vi "Read XML HW Configuration File_Parse Channels.vi"(8 "error in (no error)":errorcluster, 11 "channel429":refnum<k24>[](array[refnum])) -> (0 "error out":errorcluster, 3 "Array":T1[](array[typedef]) {"speed" items=["Auto", "Low", "High"]; "Labels"."scheduleBuildUnit" items=["Millisecond", "Microsecond"]})   [LabVIEW 2020]
doc: "This VI parses the XML HW DB."
uses:
  Controls/Ballard_Channel.ctl
  Controls/Ballard_Label.ctl
  Controls/Ballard_Word.ctl
  Controls/ARINCParam.ctl
  Shared/Controls and Global/TransferType.ctl
  Controls/Channel_direction.ctl
  Controls/Channel Speed.ctl
  C:/git/Ballard-Arinc-429-Custom-Device/Source/System Explorer/SubVIs/Parse XML Ballard/1.2/BTIXML_SerDes.dll
  1.2/BTIXML_SerDes.dll
  Ballard Arinc-429 System Explorer.lvlib
  Shared/Ballard Arinc-429 Shared.lvlib
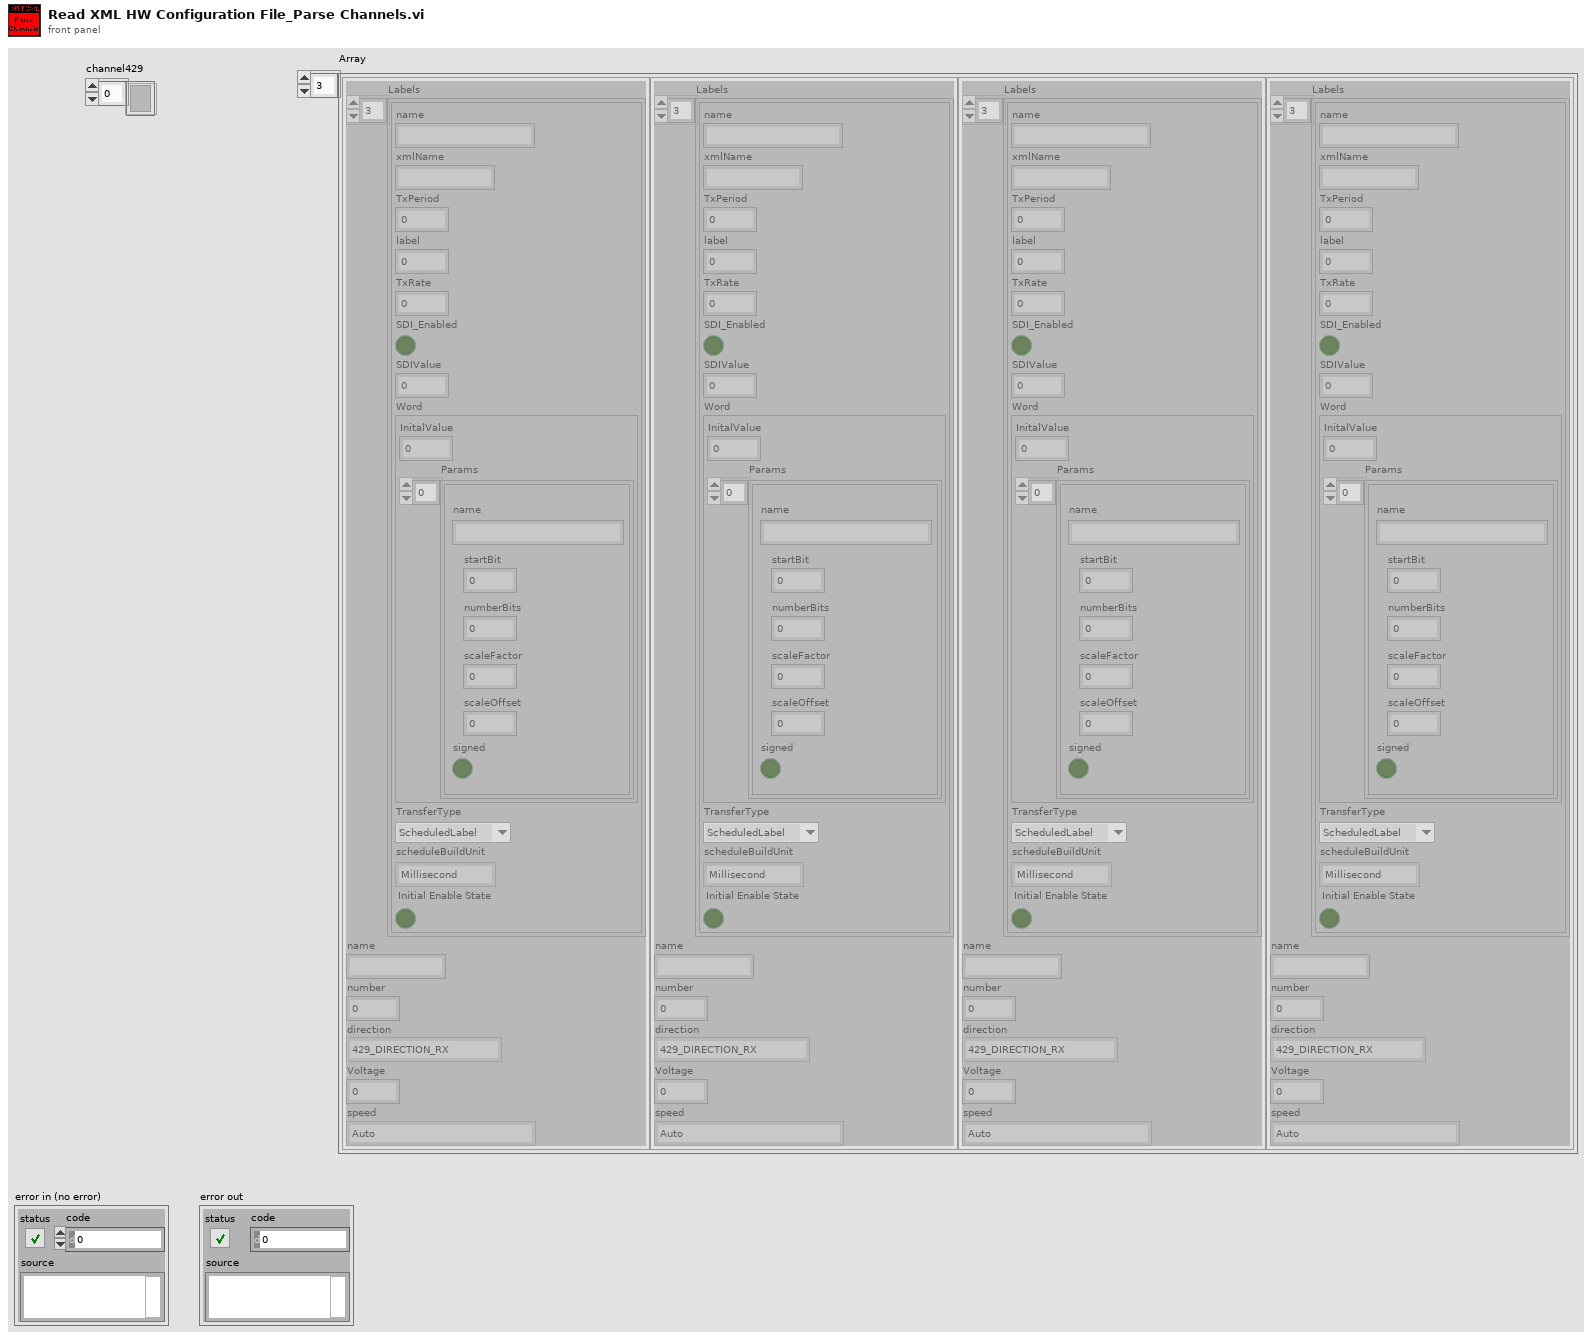
[diagram p1: front panel]
types:
  T1 = typedef "Ballard Arinc-429 System Explorer.lvlib/Ballard_Channel.ctl" = cluster{"Labels":T2[], "name":string, "number":u8, "direction":T6, "Voltage":dbl, "speed":T7}
  T2 = typedef "Ballard Arinc-429 System Explorer.lvlib/Ballard_Label.ctl" = cluster{"name":string, "xmlName":string, "TxPeriod":u32, "label":u32, "TxRate":dbl, "SDI_Enabled":bool, "SDIValue":u8, "Word":T3, "TransferType":T5, "scheduleBuildUnit":i32, "Initial Enable State":bool}
  T3 = typedef "Ballard Arinc-429 System Explorer.lvlib/Ballard_Word.ctl" = cluster{"InitalValue":u32, "Params":T4[]}
  T4 = typedef "Ballard Arinc-429 System Explorer.lvlib/ARINCParam.ctl" = cluster{"name":string, "startBit":i32, "numberBits":i32, "scaleFactor":dbl, "scaleOffset":dbl, "signed":bool}
  T5 = typedef "Ballard Arinc-429 Shared.lvlib/TransferType.ctl" = enum16{"ScheduledLabel", "Acyclic", "Block", "Strobe"}
  T6 = typedef "Ballard Arinc-429 System Explorer.lvlib/Channel_direction.ctl" = enum16{"429_DIRECTION_RX", "429_DIRECTION_TX"}
  T7 = typedef "Ballard Arinc-429 System Explorer.lvlib/Channel Speed.ctl" = i32
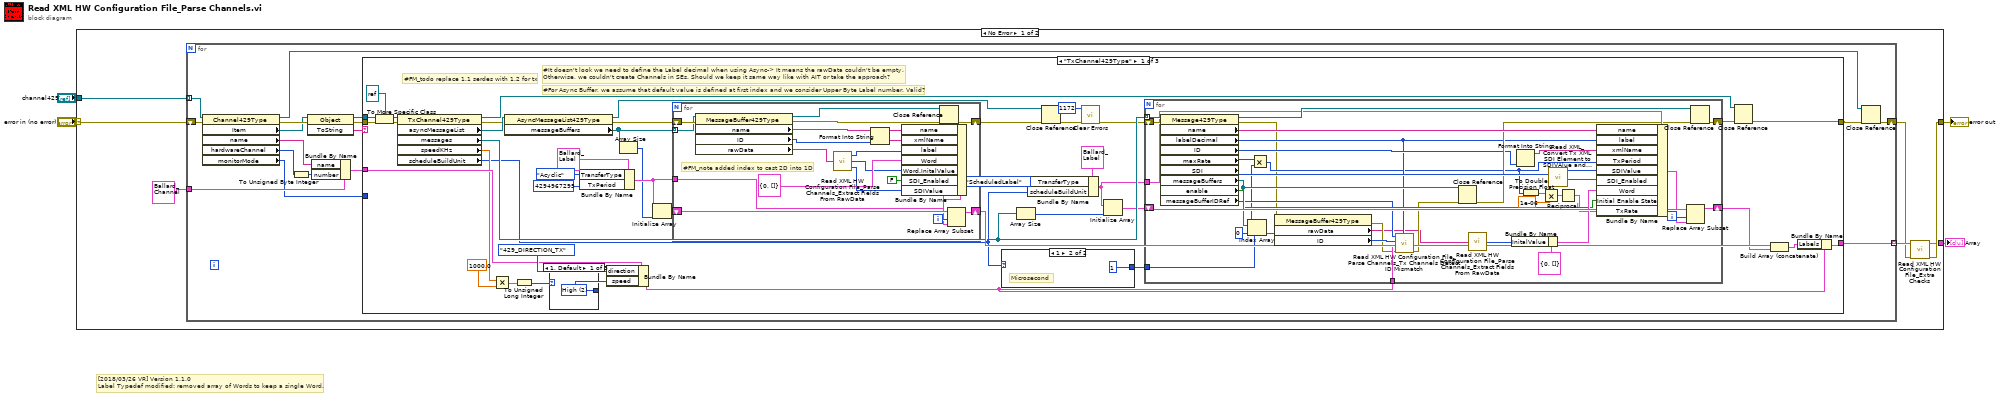
[diagram p0: block diagram]
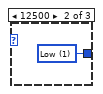
[diagram p2: hidden frame]
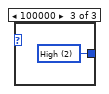
[diagram p3: hidden frame]
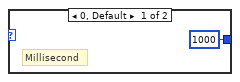
[diagram p4: hidden frame]
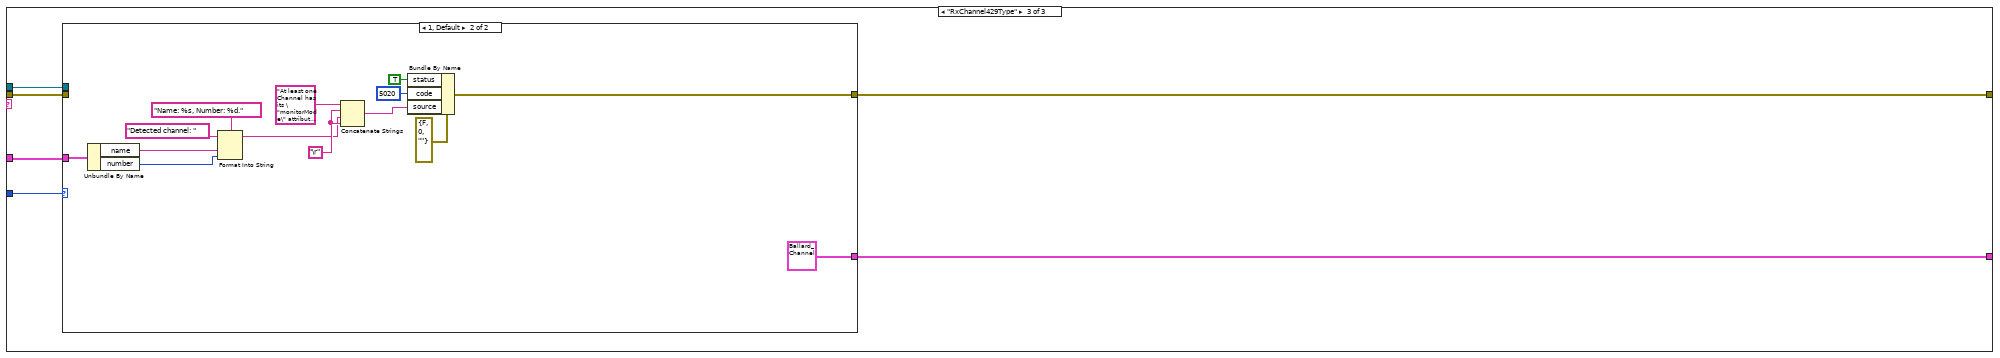
[diagram p6: hidden frame]
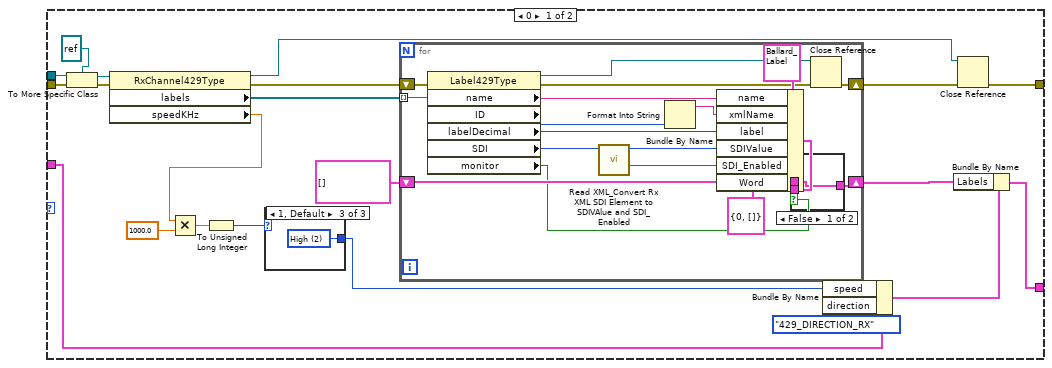
[diagram p7: hidden frame]
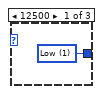
[diagram p8: hidden frame]
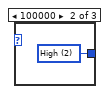
[diagram p9: hidden frame]
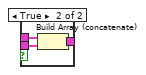
[diagram p10: hidden frame]
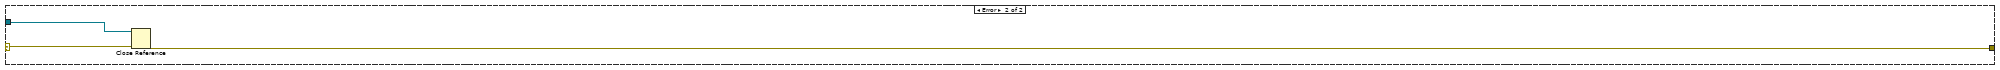
[diagram p11: hidden frame]
diagram:
  # "[2018/03/26 VR] Version 1.1.0\nLabel Typedef modified: removed array of Words to keep a single Word."
  n1 = case shown="No Error" "error in (no error)" {
    selector: "error in (no error)" -> [w9 w203]
    tunnel: [w5 _] -> w4
    tunnel: [w6 w202] -> w3
    tunnel: "channel429" -> [w10 w204]
    frame No Error {
      n2 = for {
        tunnel: w10 -> [w28] mode=indexing
        shift-right: [w16] -> w7
        shift-left: w9 -> [w25]
        tunnel: T1 {"Labels"=[], "name"="", "number"=0, "direction"=enum."429_DIRECTION_RX", "Voltage"=0.0, "speed"=0} ("channel") -> [w21]
        tunnel: [w12] -> w8 mode=indexing
        n3 = property class="Channel429Type"(reference=w28, error in=w25) -> (reference out=w15:refnum<k24>, error out=w24:errorcluster, "Item"=w22:refnum<k24>, "name"=w20:string, "hardwareChannel"=w19:i32, "monitorMode"=w14:i32)
        n4 = To Unsigned Byte Integer(number=w19) -> (unsigned 8bit integer=w18:u8)
        n5 = invoke class="Object" method="ToString"(reference=w22, error in=w24) -> (reference out=w26:refnum<k24>, error out=w23:errorcluster, "ToString"=w27:string)  [unwired: 1 in]
        n6 = Bundle By Name(cluster=w21, "name"=w20, "number"=w18) -> (w17:T1)
        n7 = case shown="\"TxChannel429Type\"" w27 {
          tunnel: w26 -> [w71 _ w141]
          tunnel: w23 -> [w70 w135 w140]
          tunnel: [w59 w135 w137] -> w13
          tunnel: w17 -> [w57 w134 w138]
          tunnel: [w46 w134 w139] -> w12
          tunnel: w14 -> [_ _ w136]
          frame "TxChannel429Type" {
            # "#FM_todo replace 1.1 serdes with 1.2 for tx"
            # "#For Async Buffer, we assume that default value is defined at first index and we consider Upper Byte Label number. Valid?"
            # "#It doesn't look we need to define the Label decimal when using Async-> It means the rawData couldn't be empty.\nOtherwise, we couldn't create Channels in SEs. Should we keep it same way like with AIT or take the approach?"
            n8 = To More Specific Class(target class=refnum<k24> refnum (".NET Refnum"), reference=w71, error in=w70) -> (specific class reference=w68:refnum<k24>, error out=w69:errorcluster)
            n9 = property class="TxChannel429Type"(reference=w68, error in=w69) -> (reference out=w60:refnum<k24>, error out=w66:errorcluster, "asyncMessageList"=w67:refnum<k24>, "messages"=w44:refnum<k24>[], "speedKHz"=w39:dbl, "scheduleBuildUnit"=w31:i32)
            n10 = Multiply(x=w39, y=1000.0) -> (x*y=w40:dbl)
            n11 = property class="AsyncMessageList429Type"(reference=w67, error in=w66) -> (reference out=w62:refnum<k24>, error out=w65:errorcluster, "messageBuffers"=w53:refnum<k24>[])
            n12 = To Unsigned Long Integer(number=w40) -> (unsigned 32bit integer=w37:u32)
            n13 = case shown="1, Default" w37 {
              tunnel: [w72 w73 w74] -> w36
              frame 1, Default {
                w72 = T7 2 items=["Auto", "Low", "High"] ("speed")
              }
              frame 12500 {
                w73 = T7 1 items=["Auto", "Low", "High"] ("speed")
              }
              frame 100000 {
                w74 = T7 2 items=["Auto", "Low", "High"] ("speed")
              }
            }
            n14 = Bundle By Name(cluster=T2 {"name"="", "xmlName"="", "TxPeriod"=0, "label"=0, "TxRate"=0.0, "SDI_Enabled"=FALSE, "SDIValue"=0, "Word"={"InitalValue"=0, "Params"=[]}, "TransferType"=enum."ScheduledLabel", "scheduleBuildUnit"=0, "Initial Enable State"=FALSE} ("Label"), "TransferType"=TransferType."Acyclic", "TxPeriod"=u32 4294967295) -> (w54:T2)
            n15 = Bundle By Name(cluster=w57, "direction"=Channel_direction."429_DIRECTION_TX", "speed"=w36) -> (w32:T1)
            n16 = Array Size(array=w53) -> (size(s)=w52:i32)
            n17 = Initialize Array(w54, w52) -> (w51:T2[])
            n18 = for {
              tunnel: w53 -> [w83] mode=indexing
              shift-right: [w93] -> w64
              shift-left: w65 -> [w84]
              tunnel: w54 -> [w88]
              shift-right: [w91] -> w49
              shift-left: w51 -> [w92]
              i -> [w90]
              # "#FM_note added index to cast 2D into 1D"
              n19 = property class="MessageBuffer429Type"(reference=w83, error in=w84) -> (reference out=w82:refnum<k24>, error out=w79:errorcluster, "name"=w81:string, "ID"=w80:i32, "rawData"=w78:string[])
              n20 = call "Read XML HW Configuration File_Parse Channels_Extract Fields From RawData.vi"("rawData"=w78) -> ("label"=w75:u32, "Word.InitialValue"=w77:u32, "SDIValue"=w76:u8)
              n21 = Format Into String(w80) -> (resulting string=w87:string)  [unwired: 3 in, 1 out]
              n22 = Bundle By Name(cluster=w88, "name"=w81, "xmlName"=w87, "label"=w75, "Word"=T3 {"InitalValue"=0, "Params"=[]}, "Word.InitalValue"=w77, "SDI_Enabled"=FALSE, "SDIValue"=w76) -> (w89:T2)
              n23 = Close Reference(reference=w82, error in (no error)=w79) -> (error out=w93:errorcluster)
              n24 = Replace Array Subset(array=w92, new element=w89, index=w90) -> (w91:T2[])
            }
            n25 = case shown="1" w31 {
              tunnel: [1000 1] -> w30
              frame 0, Default {
                # "Millisecond"
              }
              frame 1 {
                # "Microsecond"
              }
            }
            n26 = Array Size(array=w44) -> (size(s)=w42:i32)
            n27 = Bundle By Name(cluster=T2 {"name"="", "xmlName"="", "TxPeriod"=0, "label"=0, "TxRate"=0.0, "SDI_Enabled"=FALSE, "SDIValue"=0, "Word"={"InitalValue"=0, "Params"=[]}, "TransferType"=enum."ScheduledLabel", "scheduleBuildUnit"=0, "Initial Enable State"=FALSE} ("Label"), "TransferType"=TransferType."ScheduledLabel", "scheduleBuildUnit"=w31) -> (w43:T2)
            n28 = Close Reference(reference=w62, error in (no error)=w64) -> (error out=w63:errorcluster)
            n29 = call <vilib>:"Clear Errors.vi"("error in (no error)"=w63, "specific error code to clear (0: all)"=1172) -> ("error out"=w34:errorcluster)  [unwired: 4 in, 1 out]
            n30 = Initialize Array(w43, w42) -> (w41:T2[])
            n31 = for {
              tunnel: w44 -> [w133] mode=indexing
              shift-right: [w131] -> w61
              shift-left: w34 -> [w132]
              tunnel: w43 -> [w126]
              shift-right: [w129] -> w35
              shift-left: w41 -> [w127]
              tunnel: w32 -> [w112]
              tunnel: w30 -> [w108]
              i -> [w128]
              n32 = property class="Message429Type"(reference=w133, error in=w132) -> (reference out=w130:refnum<k24>, error out=w100:errorcluster, "name"=w125:string, "labelDecimal"=w110:i32, "ID"=w113:i32, "maxRate"=w109:i32, "SDI"=w122:i32, "messageBuffers"=w118:refnum<k24>[], "enable"=w114:bool, "messageBufferIDRef"=w111:i32)
              n33 = Index Array(array=w118, index=0) -> (element=w101:refnum<k24>)
              n34 = Multiply(x=w109, y=w108) -> (x*y=w107:i32)
              n35 = property class="MessageBuffer429Type"(reference=w101, error in=w100) -> (error out=w99:errorcluster, "rawData"=w97:string[], "ID"=w102:i32)  [unwired: 1 out]
              n36 = call "Read XML HW Configuration File_Parse Channels_Tx Channels Detect ID Mismatch.vi"("Label"=w110, "error in (no error)"=w99, "channel"=w112, "messageBuffer ID"=w102, "messageBufferIDRef"=w111) -> ("error out"=w98:errorcluster)  [unwired: 6 in]
              n37 = Close Reference(reference=w118, error in (no error)=w98) -> (error out=w117:errorcluster)
              n38 = call "Read XML HW Configuration File_Parse Channels_Extract Fields From RawData.vi"("rawData"=w97) -> ("Word.InitialValue"=w96:u32)  [unwired: 2 out]
              n39 = Bundle By Name(cluster=T3 {"InitalValue"=0, "Params"=[]} ("Word"), "InitalValue"=w96) -> (w115:T3)
              n40 = Format Into String(w113) -> (resulting string=w123:string)  [unwired: 3 in, 1 out]
              n41 = To Double Precision Float(number=w107) -> (double precision float=w106:dbl)
              n42 = Multiply(x=w106, y=1e-06) -> (x*y=w104:dbl)
              n43 = call "Read XML_Convert Tx XML SDI Element to SDIVAlue and SDI_Enabled.vi"("SDI"=w122) -> ("SDI_Enabled"=w120:bool, "SDIValue"=w121:u8)  [unwired: 9 in]
              n44 = Reciprocal(x=w104) -> (1/x=w103:dbl)
              n45 = Bundle By Name(cluster=w126, "name"=w125, "label"=w110, "xmlName"=w123, "TxPeriod"=w107, "SDIValue"=w121, "SDI_Enabled"=w120, "Word"=w115, "Initial Enable State"=w114, "TxRate"=w103) -> (w124:T2)
              n46 = Replace Array Subset(array=w127, new element=w124, index=w128) -> (w129:T2[])
              n47 = Close Reference(reference=w130, error in (no error)=w117) -> (error out=w131:errorcluster)
            }
            n48 = Close Reference(reference=w60, error in (no error)=w61) -> (error out=w59:errorcluster)
            n49 = Build Array (concatenate)(w49, w35) -> (w45:T2[])
            n50 = Bundle By Name(cluster=w32, "Labels"=w45) -> (w46:T1)
          }
          frame "False", Default {
          }
          frame "RxChannel429Type" {
            n51 = case shown="1, Default" w136 {
              tunnel: w141 -> [w162 _]
              tunnel: w140 -> [w161 _]
              tunnel: [w154 T1 {"Labels"=[], "name"="", "number"=0, "direction"=enum."429_DIRECTION_RX", "Voltage"=0.0, "speed"=0} ("channel")] -> w139
              tunnel: w138 -> [w152 w193]
              tunnel: [w149 w197] -> w137
              frame 0 {
                n52 = To More Specific Class(target class=refnum<k24> refnum (".NET Refnum"), reference=w162, error in=w161) -> (specific class reference=w159:refnum<k24>, error out=w160:errorcluster)
                n53 = property class="RxChannel429Type"(reference=w159, error in=w160) -> (reference out=w148:refnum<k24>, error out=w157:errorcluster, "labels"=w158:refnum<k24>[], "speedKHz"=w145:dbl)
                n54 = Multiply(x=w145, y=1000.0) -> (x*y=w147:dbl)
                n55 = To Unsigned Long Integer(number=w147) -> (unsigned 32bit integer=w144:u32)
                n56 = case shown="1, Default" w144 {
                  tunnel: [w163 w164 w165] -> w143
                  frame 12500 {
                    w163 = T7 1 items=["Auto", "Low", "High"] ("speed")
                  }
                  frame 100000 {
                    w164 = T7 2 items=["Auto", "Low", "High"] ("speed")
                  }
                  frame 1, Default {
                    w165 = T7 2 items=["Auto", "Low", "High"] ("speed")
                  }
                }
                n57 = for {
                  tunnel: w158 -> [w183] mode=indexing
                  shift-right: [w172] -> w150
                  shift-left: w157 -> [w182]
                  shift-right: [w180] -> w153
                  shift-left: T2[] [] ("Labels") -> [w181]
                  n58 = property class="Label429Type"(reference=w183, error in=w182) -> (reference out=w171:refnum<k24>, error out=w173:errorcluster, "name"=w175:string, "ID"=w176:i32, "labelDecimal"=w178:i32, "SDI"=w170:i32, "monitor"=w167:bool)
                  n59 = call "Read XML_Convert Rx XML SDI Element to SDIVAlue and SDI_Enabled.vi"("SDI"=w170) -> ("SDI_Enabled"=w168:bool, "SDIValue"=w169:u8)  [unwired: 9 in]
                  n60 = Format Into String(w176) -> (resulting string=w177:string)  [unwired: 3 in, 1 out]
                  n61 = Bundle By Name(cluster=T2 {"name"="", "xmlName"="", "TxPeriod"=0, "label"=0, "TxRate"=0.0, "SDI_Enabled"=FALSE, "SDIValue"=0, "Word"={"InitalValue"=0, "Params"=[]}, "TransferType"=enum."ScheduledLabel", "scheduleBuildUnit"=0, "Initial Enable State"=FALSE} ("TxScheduledLabel"), "name"=w175, "xmlName"=w177, "label"=w178, "SDIValue"=w169, "SDI_Enabled"=w168, "Word"=T3 {"InitalValue"=0, "Params"=[]}) -> (w174:T2)
                  n62 = case shown="False" w167 {
                    tunnel: w181 -> [w184 w187]
                    tunnel: [w184 w186] -> w180
                    tunnel: w174 -> [_ w185]
                    frame False {
                    }
                    frame True {
                      n63 = Build Array (concatenate)(w187, w185) -> (w186:T2[])
                    }
                  }
                  n64 = Close Reference(reference=w171, error in (no error)=w173) -> (error out=w172:errorcluster)
                }
                n65 = Bundle By Name(cluster=w152, "speed"=w143, "direction"=Channel_direction."429_DIRECTION_RX") -> (w155:T1)
                n66 = Bundle By Name(cluster=w155, "Labels"=w153) -> (w154:T1)
                n67 = Close Reference(reference=w148, error in (no error)=w150) -> (error out=w149:errorcluster)
              }
              frame 1, Default {
                w192 = "\r"
                n68 = Unbundle By Name(w193) -> ("name"=w191:string, "number"=w190:u8)
                n69 = Format Into String(format string="Name: %s, Number: %d.", initial string="Detected channel: ", w191, w190) -> (resulting string=w189:string)  [unwired: 1 in, 1 out]
                n70 = Concatenate Strings("At least one Channel has its \"monitorMode\" attribute set to \"All\" which is not supported. Only \"Selective\" value (default value) is supported for this attribute.", w192, w189, w192) -> (w198:string)
                n71 = Bundle By Name(cluster=errorcluster {"status"=FALSE, "code"=0, "source"=""} ("error in (no error) 2"), "status"=TRUE, "code"=5020, "source"=w198) -> (w197:errorcluster)
              }
            }
          }
        }
        n72 = Close Reference(reference=w15, error in (no error)=w13) -> (error out=w16:errorcluster)
      }
      n73 = call "Read XML HW Configuration File_Extra Checks.vi"("error in (no error)"=w7, "Array In"=w8) -> ("error out"=w6:errorcluster, "Array Out"=w5:T1[])  [unwired: 8 in]
    }
    frame Error {
      n74 = Close Reference(reference=w204, error in (no error)=w203) -> (error out=w202:errorcluster)
    }
  }
  "Array" <- w4
  "error out" <- w3
